vi "CANShark_SetBaudrate.vi"(9 "BaudRate":i32, 10 "Device Handler":i64, 11 "error in (no error)":errorcluster) -> (2 "CAN BaudRate":u8, 3 "error out":errorcluster)   [LabVIEW 2026]
uses:
  x64/Release/CanSharkApi_Dll1.dll
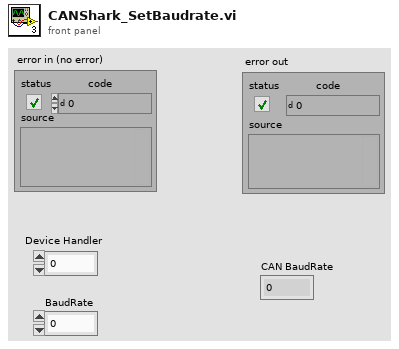
[diagram p1: front panel]
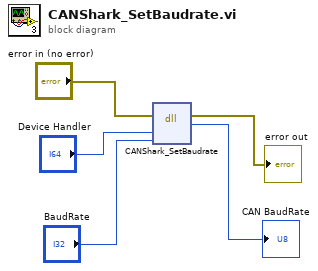
[diagram p0: block diagram]
diagram:
  n1 = dll-call lib="C:/Users/TECQNIO/Documents/CANSHARK LABVIEW API PACKAGE/x64/Release/CanSharkApi_Dll1.dll" fn="CANShark_SetBaudrate"(error in="error in (no error)", "device"="Device Handler", "BaudRate"="BaudRate") -> (error out=→"error out":errorcluster, "return type"=→"CAN BaudRate":u8)  [unwired: 4 in, 1 out]
